vi "Get Datalog Config path.vi"(8 "error in (no error)":errorcluster) -> (0 "error out":errorcluster, 3 "Data Log Config":path)   [LabVIEW 2018]
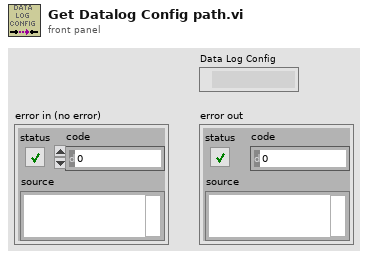
[diagram p1: front panel]
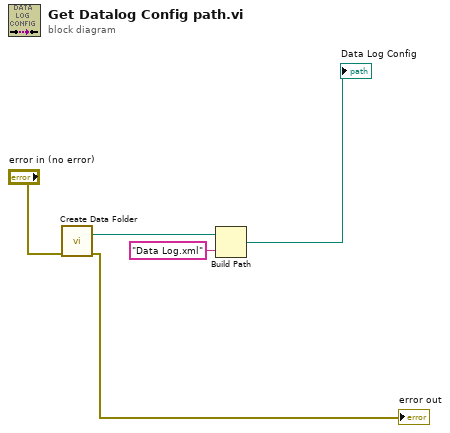
[diagram p0: block diagram]
diagram:
  n1 = call "Create Data Folder.vi"("error in (no error)"="error in (no error)") -> ("error out"=→"error out":errorcluster, "Data path"=w3:path)  [unwired: 9 in]
  n2 = Build Path(base path=w3, name or relative path="Data Log.xml") -> (appended path=→"Data Log Config":path)
